vi "Controller Request Stop.vi"(7 "Sync Objects":T3, 8 "error in (no error)":errorcluster) -> (0 "error out":errorcluster)   [LabVIEW 2011, in "Controller VIs.lvlib"]
doc: "Requests the completion of all parallel loops running in the FOFB Controller. Sends a stop notification through the \"Stop Notifier\" and forces all blocking notifiers to be released."
uses:
  Controller VIs.lvlib
  Types Definitions/Type Synchronization Objects.ctl
  Types Definitions/Type Blocking Synchronization Objects.ctl
  Types Definitions/Type FA Request Parameters.ctl
  Types Definitions/Type BPM and PS select cluster.ctl
  Types Definitions/Type FA File Parameters.ctl
  Types Definitions/Type Monitoring Data.ctl
  Types Definitions/Type Diagnostics Data.ctl
  Types Definitions/Type CPU Loads Array.ctl
  Types Definitions/Type CPU Loads.ctl
  Types Definitions/Type Non-blocking Synchronization Objects.ctl
  Types Definitions/Type FOFB Variables.ctl
  Types Definitions/Type Actuation State.ctl
  Misc VIs.lvlib
  Type Definitions.lvlib
panel:
  out "Blocking":T1
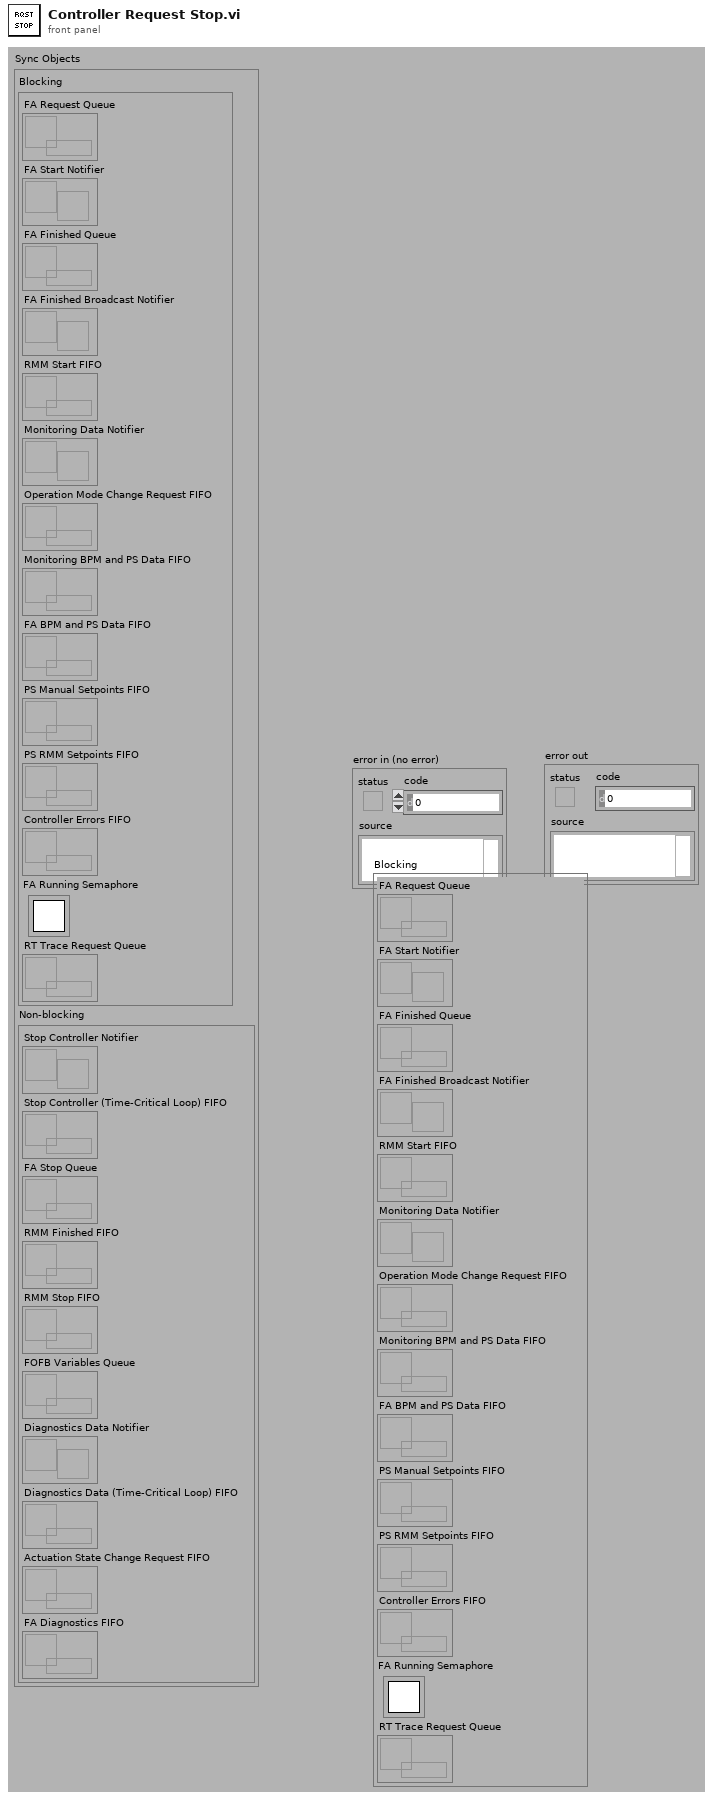
[diagram p1: front panel]
types:
  T1 = typedef "Type Definitions.lvlib/Type Blocking Synchronization Objects.ctl" = cluster{"FA Request Queue":refnum<queue>, "FA Start Notifier":refnum<notifier>, "FA Finished Queue":refnum<queue>, "FA Finished Broadcast Notifier":refnum<notifier>, "RMM Start FIFO":refnum<k33>, "Monitoring Data Notifier":refnum<notifier>, "Operation Mode Change Request FIFO":refnum<k33>, "Monitoring BPM and PS Data FIFO":refnum<k33>, "FA BPM and PS Data FIFO":refnum<k33>, "PS Manual Setpoints FIFO":refnum<k33>, "PS RMM Setpoints FIFO":refnum<k33>, "Controller Errors FIFO":refnum<k33>, "FA Running Semaphore":T2, "RT Trace Request Queue":refnum<queue>}
  T2 = typedef "Semaphore RefNum" = refnum<k1>
  T3 = typedef "Type Definitions.lvlib/Type Synchronization Objects.ctl" = cluster{"Blocking":T1, "Non-blocking":T4}
  T4 = typedef "Type Definitions.lvlib/Type Non-blocking Synchronization Objects.ctl" = cluster{"Stop Controller Notifier":refnum<notifier>, "Stop Controller (Time-Critical Loop) FIFO":refnum<k33>, "FA Stop Queue":refnum<queue>, "RMM Finished FIFO":refnum<k33>, "RMM Stop FIFO":refnum<k33>, "FOFB Variables Queue":refnum<queue>, "Diagnostics Data Notifier":refnum<notifier>, "Diagnostics Data (Time-Critical Loop) FIFO":refnum<k33>, "Actuation State Change Request FIFO":refnum<k33>, "FA Diagnostics FIFO":refnum<k33>}
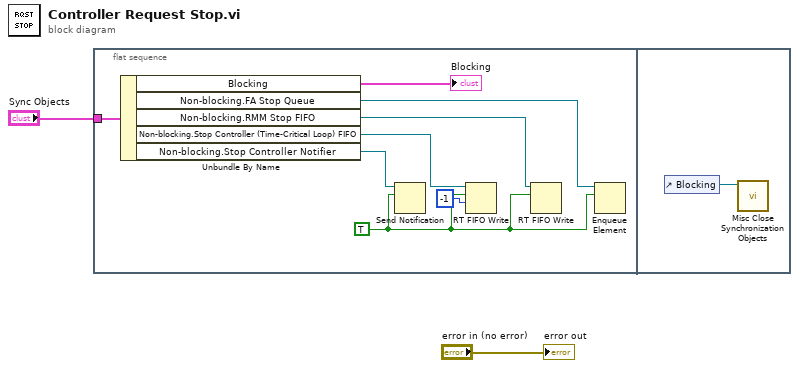
[diagram p0: block diagram]
diagram:
  n1 = flat-sequence {
    tunnel: "Sync Objects" -> [w10]
    frame #0 {
      w4 = TRUE ("notification")
      n2 = Unbundle By Name(w10) -> ("Blocking"=→"Blocking":T1, "Non-blocking.FA Stop Queue"=w9:refnum<queue>, "Non-blocking.RMM Stop FIFO"=w8:refnum<k33>, "Non-blocking.Stop Controller (Time-Critical Loop) FIFO"=w6:refnum<k33>, "Non-blocking.Stop Controller Notifier"=w7:refnum<notifier>)
      n3 = Send Notification(notification=w4, notifier=w7) -> ()  [unwired: 1 in, 2 out]
      n4 = RT FIFO Write(0:w6, 1:w4, 2:-1 ("timeout in ms (0)")) -> ()  [unwired: 2 in, 4 out]
      n5 = RT FIFO Write(0:w8, 1:w4) -> ()  [unwired: 3 in, 4 out]
      n6 = Enqueue Element(queue=w9, element=w4) -> ()  [unwired: 2 in, 3 out]
    }
    frame #1 {
      n7 = control-ref of="Blocking"() -> (w11:refnum<vi>)
      n8 = call "Misc Close Synchronization Objects.vi"("Cluster Reference"=w11) -> ()  [unwired: 10 in, 1 out]
    }
  }
  "error out" <- "error in (no error)"
